vi "Update.vi"(8 "error in (no error)":errorcluster, 10 "Model in":refnum<class "Model.lvclass">, 11 "Enabled State in":refnum<class "Enabled State.lvclass">) -> (0 "error out":errorcluster, 2 "Model out":refnum<class "Model.lvclass">, 3 "Enabled State out":refnum<class "Enabled State.lvclass">)   [LabVIEW 2015, in "Enabled State.lvclass"]
uses:
  Enabled State.lvclass
  Model/Model/Model.lvclass
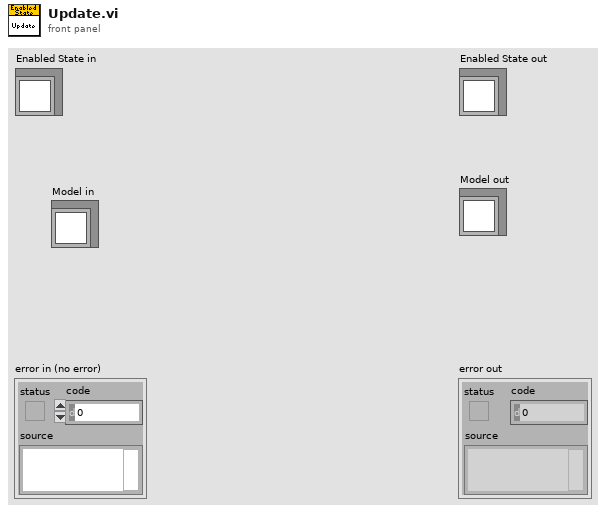
[diagram p1: front panel]
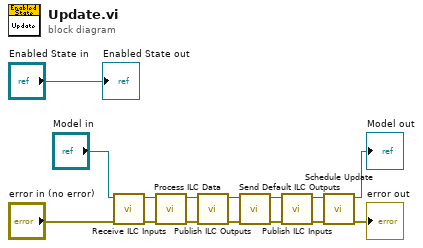
[diagram p0: block diagram]
diagram:
  n1 = call "Receive ILC Inputs.vi"("error in (no error)"="error in (no error)", "Model in"="Model in") -> ("error out"=w1:errorcluster, "Model out"=w2:refnum<class "Model.lvclass">)  [unwired: 8 in]
  n2 = call "Process ILC Data.vi"("error in (no error)"=w1, "Model in"=w2) -> ("error out"=w7:errorcluster, "Model out"=w13:refnum<class "Model.lvclass">)  [unwired: 8 in]
  n3 = call "Publish ILC Outputs.vi"("error in (no error)"=w7, "Model in"=w13) -> ("error out"=w6:errorcluster, "Model out"=w12:refnum<class "Model.lvclass">)  [unwired: 8 in]
  n4 = call "Send Default ILC Outputs.vi"("error in (no error)"=w6, "Model in"=w12) -> ("error out"=w5:errorcluster, "Model out"=w11:refnum<class "Model.lvclass">)  [unwired: 8 in]
  n5 = call "Publish ILC Inputs.vi"("error in (no error)"=w5, "Model in"=w11) -> ("error out"=w4:errorcluster, "Model out"=w10:refnum<class "Model.lvclass">)  [unwired: 8 in]
  n6 = call "Schedule Update.vi"("error in (no error)"=w4, "Model in"=w10) -> ("error out"=→"error out":errorcluster, "Model out"=→"Model out":refnum<class "Model.lvclass">)  [unwired: 8 in]
  "Enabled State out" <- "Enabled State in"
